vi "confocal3D.vi"() -> ()   [LabVIEW 2025]
uses:
  <vilib>/Analysis/1siggen.llb/Ramp Pattern by Samples.vi
  <vilib>/DAQmx/create/channels.llb/DAQmx Create Channel (AO-Voltage-Basic).vi
  <vilib>/DAQmx/configure/timing.llb/DAQmx Timing (Sample Clock).vi
  <vilib>/DAQmx/miscellaneous.llb/DAQmx Fill In Error Info.vi
  <vilib>/DAQmx/configure/events/hardwareSignals.llb/DAQmx Export Signal (Most Signals).vi
  <vilib>/DAQmx/read.llb/DAQmx Read (Counter 1D U32 1Chan NSamp).vi
  <vilib>/DAQmx/create/channels.llb/DAQmx Create Channel (CI-Count Edges).vi
  <vilib>/DAQmx/write.llb/DAQmx Write (Analog 1D Wfm NChan NSamp).vi
  <vilib>/DAQmx/write.llb/DAQmx Write (Analog DBL 1Chan 1Samp).vi
  <vilib>/Analysis/NI_AALBase.lvlib
panel:
  in  "step-size in microns(depth)":dbl=0.1428 format="%#_13g"
  in  "Path":path
  in  "Number of slices":i32
  in  "Enter length (nm)":dbl
  out "64bit integer":i64[](array[numeric])
  in  "pixels":dbl
  out "transposed array":dbl[][](array[numeric])
  out "Intensity Graph":dbl[][](graph)
  out "Min Voltage (V)":dbl
  out "Max Voltage (V)":dbl
  in  "Dwell time (s)":dbl
  in  "Sample mode":i32(ring)=10178 items=["Finite Samples"=10178, "Continuous Samples"=10123, "Hardware Timed Single Point"=12522]
  out "appended array":dbl[][](array[numeric])
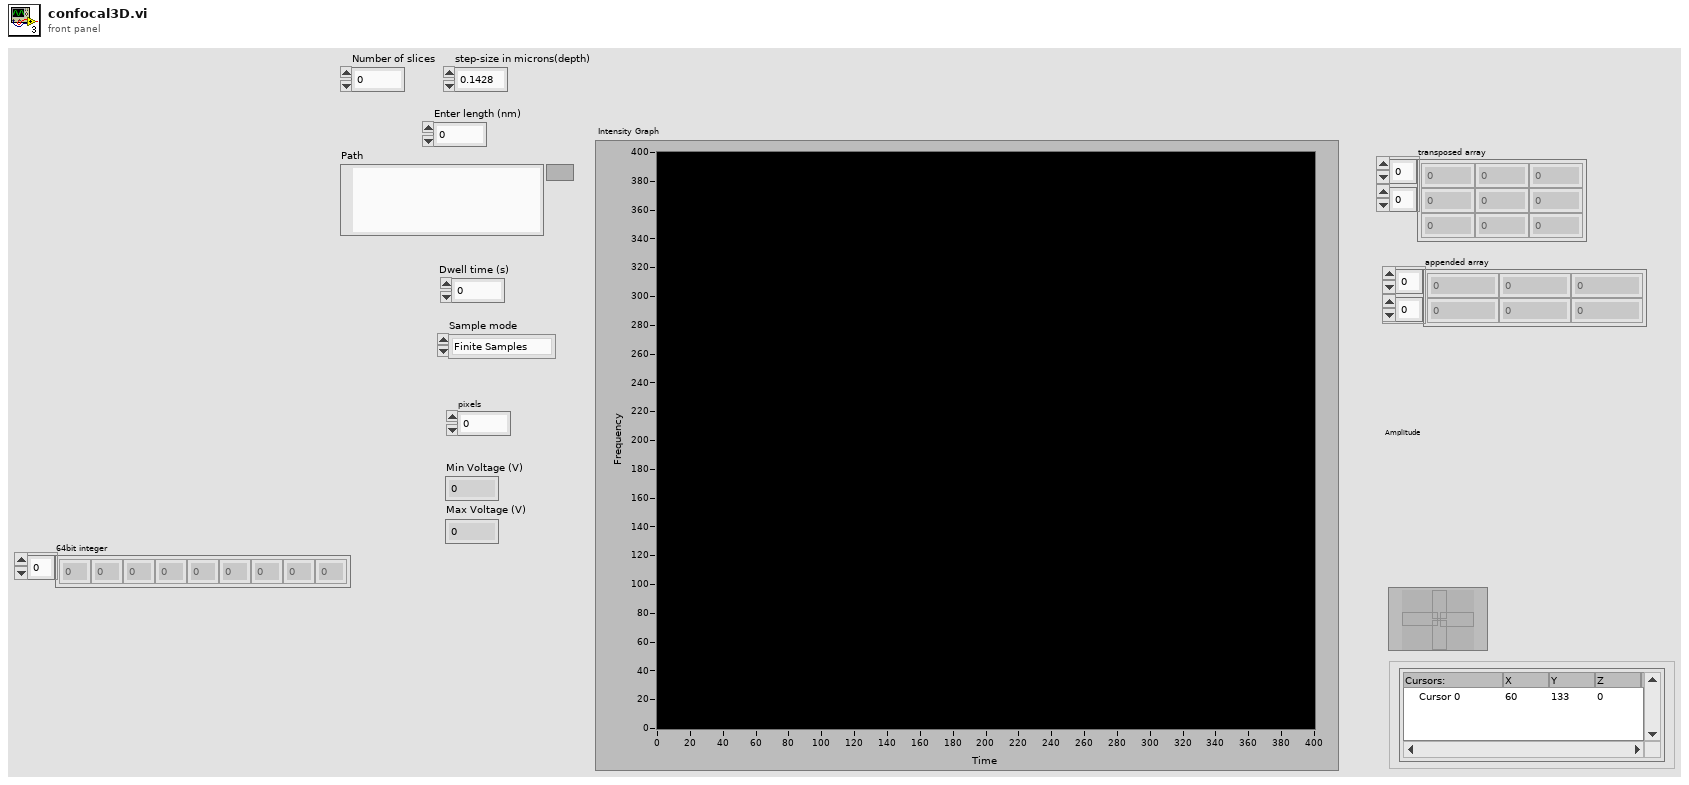
[diagram p1: front panel]
types:
  T1 = enum16{"big-endian, network order", "native, host order", "little-endian"}
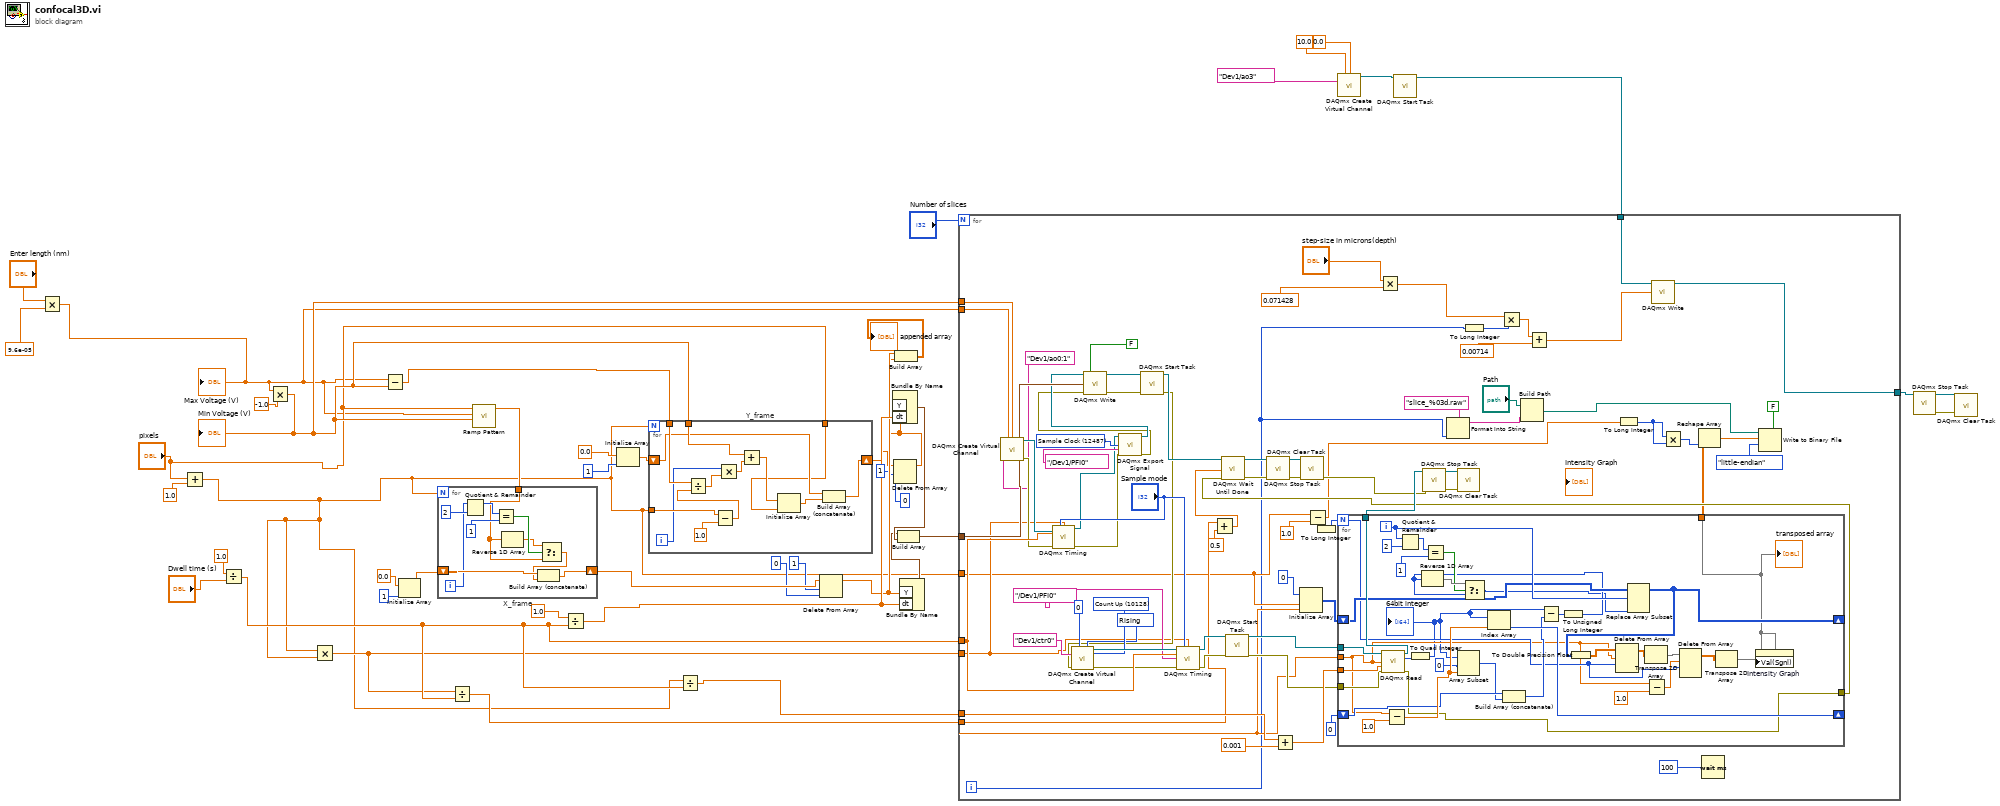
[diagram p0: block diagram]
diagram:
  n1 = Multiply(x="Enter length (nm)", y=9.6e-05) -> (x*y=w4:dbl)
  "Max Voltage (V)" <- w4
  n2 = Add(x="pixels", y=1.0) -> (x+y=w14:dbl)
  n3 = Divide(x=1.0, y="Dwell time (s)") -> (x/y=w21:dbl)
  n4 = Multiply(x=w4, y=-1.0) -> (x*y=w16:dbl)
  "Min Voltage (V)" <- w16
  n5 = Multiply(x=w14, y=w14) -> (x*y=w19:dbl)
  n6 = Subtract(x=w4, y=w16) -> (x-y=w30:dbl)
  n7 = Initialize Array(0.0 ("element"), 1 ("dimension size")) -> (w37:dbl[])
  n8 = Divide(x=w19, y=w21) -> (x/y=w18:dbl)
  n9 = call-poly <vilib>:"Ramp Pattern.vi"("start"=w16, "end"=w4, "samples"="pixels") -> ("Ramp Pattern"=w43:dbl[])  [unwired: 7 in, 1 out]
  n10 = for "X_frame" {
    N: w14 -> [_]
    shift-right: [w54] -> w29
    shift-left: w37 -> [w55]
    tunnel: w43 -> [w48]
    i -> [w49]
    n11 = Quotient & Remainder(x=w49, y=2) -> (x-y*floor(x/y)=w52:i32)  [unwired: 1 out]
    n12 = Equal?(x=w52, y=1) -> (x = y?=w50:bool)
    n13 = Reverse 1D Array(array=w48) -> (reversed array=w47:dbl[])
    n14 = Select(t=w47, s=w50, f=w48) -> (s? t:f=w46:dbl[])
    n15 = Build Array (concatenate) "Build Array"(w55, w46) -> (w54:dbl[])
  }
  n16 = Divide(x=1.0, y=w21) -> (x/y=w39:dbl)
  n17 = Initialize Array(0.0 ("element"), 1 ("dimension size")) -> (w38:dbl[])
  n18 = for "Y_frame" {
    N: w14 -> [_]
    tunnel: w14 -> [w68]
    tunnel: w30 -> [w66]
    tunnel: w16 -> [w61]
    tunnel: "pixels" -> [w56]
    shift-right: [w57] -> w25
    shift-left: w38 -> [w58]
    i -> [w63]
    n19 = Subtract(x=w68, y=1.0) -> (x-y=w65:dbl)
    n20 = Divide(x=w66, y=w65) -> (x/y=w64:dbl)
    n21 = Multiply(x=w63, y=w64) -> (x*y=w62:dbl)
    n22 = Add(x=w61, y=w62) -> (x+y=w60:dbl)
    n23 = Initialize Array(w60, w56) -> (w59:dbl[])
    n24 = Build Array (concatenate)(w58, w59) -> (w57:dbl[])
  }
  n25 = Divide(x=w14, y=w21) -> (x/y=w20:dbl)
  n26 = Delete From Array "Delete From Array"(array=w29, length=1, index=0) -> (array with subset deleted=w26:dbl[])  [unwired: 1 out]
  n27 = Delete From Array "Delete From Array"(array=w25, length=1, index=0) -> (array with subset deleted=w22:dbl[])  [unwired: 1 out]
  n28 = Bundle By Name("Y"=w22, "dt"=w39) -> (w41:waveform(dbl))  [unwired: 1 in]
  n29 = Build Array(w26, w22) -> (→"appended array":dbl[][])
  n30 = Bundle By Name("Y"=w26, "dt"=w39) -> (w40:waveform(dbl))  [unwired: 1 in]
  n31 = Build Array(w40, w41) -> (w42:waveform(dbl)[])
  n32 = call-poly <vilib>:"DAQmx Create Virtual Channel.vi"("maximum value"=10.0, "minimum value"=0.0, "physical channels"=tag "Dev1/ao3") -> ("task out"=w12:refnum<k21>)  [unwired: 11 in, 1 out]
  n33 = call <vilib>:"DAQmx Start Task.vi"("task/channels in"=w12) -> ("task out"=w11:refnum<k21>)  [unwired: 13 in, 1 out]
  n34 = for {
    N: "Number of slices" -> [_]
    tunnel: w42 -> [w131]
    tunnel: w21 -> [w117]
    tunnel: w20 -> [w114]
    tunnel: w19 -> [w99]
    tunnel: w18 -> [w98]
    tunnel: w16 -> [w95]
    tunnel: w14 -> [w93]
    tunnel: w4 -> [w92]
    tunnel: w11 -> [w90]
    tunnel: [w89] -> w8
    i -> [w81]
    w124 = 12487 items=["AI Convert Clock"=12484, "10MHz Reference Clock"=12536, "20MHz Timebase Clock"=12486, "Sample Clock"=12487, "Advance Trigger"=12488, "Reference Trigger"=12490, "Start Trigger"=12491, "Advance Complete Event"=12492, "AI Hold Complete Event"=12493, "Counter Output Event"=12494, "Change Detection Event"=12511, "Watchdog Timer Expired Event"=12512] ("signal")
    w127 = 10280 items=["Rising"=10280, "Falling"=10171] ("edge")
    w128 = 10128 items=["Count Up"=10128, "Count Down"=10124, "Externally Controlled"=10326] ("count direction")
    n35 = call-poly <vilib>:"DAQmx Create Virtual Channel.vi"("maximum value"=w92, "minimum value"=w95, "physical channels"="Dev1/ao0:1" ("Galvo mirror path")) -> ("task out"=w130:refnum<k21>, "error out"=w112:errorcluster)  [unwired: 11 in]
    n36 = call-poly <vilib>:"DAQmx Timing.vi"("task/channels in"=w130, "sample mode"="Sample mode", "samples per channel"=w99, "rate"=w117, "error in"=w112) -> ("task out"=w122:refnum<k21>, "error out"=w111:errorcluster)  [unwired: 9 in]
    n37 = call-poly <vilib>:"DAQmx Export Signal.vi"("task/channels in"=w122, "signal"=w124, "output terminal"=tag "/Dev1/PFI0", "error in"=w111) -> ("task out"=w121:refnum<k21>, "error out"=w110:errorcluster)  [unwired: 10 in]
    n38 = call-poly <vilib>:"DAQmx Write.vi"("task/channels in"=w121, "auto start"=FALSE, "data"=w131, "error in"=w110) -> ("task out"=w132:refnum<k21>, "error out"=w109:errorcluster)  [unwired: 9 in, 1 out]
    n39 = call <vilib>:"DAQmx Start Task.vi"("task/channels in"=w132, "error in"=w109) -> ("task out"=w139:refnum<k21>, "error out"=w106:errorcluster)  [unwired: 12 in]
    n40 = call-poly <vilib>:"DAQmx Create Virtual Channel.vi"("initial count"=u32 0, "count direction"=w128, "edge"=w127, "counter"="Dev1/ctr0" ("Counter path"), "error in"=w106) -> ("task out"=w134:refnum<k21>, "error out"=w108:errorcluster)  [unwired: 9 in]
    n41 = call-poly <vilib>:"DAQmx Timing.vi"("task/channels in"=w134, "sample mode"="Sample mode", "samples per channel"=w99, "rate"=w117, "source"=tag "/Dev1/PFI0", "error in"=w108) -> ("task out"=w135:refnum<k21>, "error out"=w107:errorcluster)  [unwired: 8 in]
    n42 = Add(x=w98, y=0.5) -> (x+y=w96:dbl)
    n43 = call <vilib>:"DAQmx Start Task.vi"("task/channels in"=w135, "error in"=w107) -> ("task out"=w136:refnum<k21>, "error out"=w101:errorcluster)  [unwired: 12 in]
    n44 = Add(x=w114, y=0.001) -> (x+y=w118:dbl)
    n45 = Initialize Array(u32 0 ("element"), w93, w93) -> (w138:u32[][])
    n46 = Subtract(x=w93, y=1.0) -> (x-y=w70:dbl)
    n47 = To Long Integer(number=w70) -> (32bit integer=w82:i32)
    n48 = for {
      N: w82 -> [w149]
      tunnel: w93 -> [w146]
      tunnel: w118 -> [w176]
      tunnel: w136 -> [w175]
      shift-right: [w158] -> _
      shift-left: w138 -> [w161]
      tunnel: [w170] -> w113
      shift-right: [w167] -> _
      shift-left: u64 0 ("Numeric") -> [w165]
      tunnel: w101 -> [w156]
      tunnel: [w155] -> w100
      tunnel: [w143] -> w69
      i -> [w162]
      n49 = call-poly <vilib>:"DAQmx Read.vi"("task/channels in"=w175, "number of samples per channel"=w146, "timeout"=w176, "error in"=w156) -> ("task out"=w170:refnum<k21>, "data"=w157:u32[], "error out"=w155:errorcluster)  [unwired: 9 in]
      n50 = Subtract(x=w146, y=1.0) -> (x-y=w166:dbl)
      n51 = Quotient & Remainder(x=w162, y=2) -> (x-y*floor(x/y)=w173:i32)  [unwired: 1 out]
      n52 = To Quad Integer(1:w157) -> (0:w144:i64[])
      "64bit integer" <- w144
      n53 = Equal?(x=w173, y=1) -> (x = y?=w169:bool)
      n54 = Array Subset "Array Subset"(array=w144, index=0, length=w166) -> (w145:i64[])
      n55 = Index Array "Index Array"(array=w144, index=w166) -> (element=w167:i64)
      n56 = Build Array (concatenate) "Build Array"(w165, w145) -> (w164:u64[])
      n57 = Subtract(x=w144, y=w164) -> (x-y=w163:u64[])
      n58 = To Unsigned Long Integer(number=w163) -> (unsigned 32bit integer=w160:u32[])
      n59 = Reverse 1D Array(array=w160) -> (reversed array=w171:u32[])
      n60 = Select(t=w171, s=w169, f=w160) -> (s? t:f=w159:u32[])
      n61 = Replace Array Subset "Replace Array Subset"(array=w161, new element=w159, index (row)=w162) -> (w158:u32[][])  [unwired: 1 in]
      n62 = To Double Precision Float(number=w158) -> (double precision float=w154:dbl[][])
      n63 = Delete From Array(array=w154, length=w146, index (row)=w149) -> (array with subset deleted=w153:dbl[][])  [unwired: 1 in, 1 out]
      n64 = Transpose 2D Array(2D array=w153) -> (transposed array=w152:dbl[][])
      n65 = Subtract(x=w146, y=1.0) -> (x-y=w150:dbl)
      n66 = Delete From Array(array=w152, length=w150, index (row)=w149) -> (array with subset deleted=w148:dbl[][])  [unwired: 1 in, 1 out]
      n67 = Transpose 2D Array(2D array=w148) -> (transposed array=w143:dbl[][])
      "transposed array" <- w143
      n68 = property on="Intensity Graph" class="IntGraph (strict)"("Val(Sgnl)"=w143) -> ()  [unwired: 2 in, 2 out]
    }
    n69 = call <vilib>:"DAQmx Wait Until Done.vi"("task/channels in"=w139, "timeout (sec)"=w96, "error in"=w100) -> ("task out"=w140:refnum<k21>, "error out"=w105:errorcluster)  [unwired: 11 in]
    n70 = call <vilib>:"DAQmx Stop Task.vi"("task/channels in"=w140, "error in"=w105) -> ("task out"=w133:refnum<k21>, "error out"=w104:errorcluster)  [unwired: 12 in]
    n71 = call <vilib>:"DAQmx Clear Task.vi"("task in"=w133, "error in"=w104) -> ("error out"=w103:errorcluster)  [unwired: 13 in]
    n72 = Multiply(x="step-size in microns(depth)", y=0.071428) -> (x*y=w77:dbl)
    n73 = call <vilib>:"DAQmx Stop Task.vi"("task/channels in"=w113, "error in"=w103) -> ("task out"=w141:refnum<k21>, "error out"=w102:errorcluster)  [unwired: 12 in]
    n74 = Format Into String(format string="slice_%03d.raw", w81) -> (resulting string=w83:string)  [unwired: 2 in, 1 out]
    n75 = call <vilib>:"DAQmx Clear Task.vi"("task in"=w141, "error in"=w102) -> ()  [unwired: 13 in, 1 out]
    n76 = To Long Integer(number=w81) -> (32bit integer=w80:i32)
    n77 = Multiply(x=w77, y=w80) -> (x*y=w88:dbl)
    n78 = Build Path(base path="Path", name or relative path=w83) -> (appended path=w71:path)
    n79 = Add(x=w88, y=0.00714) -> (x+y=w87:dbl)
    n80 = To Long Integer(number=w70) -> (32bit integer=w72:i32)
    n81 = call-poly <vilib>:"DAQmx Write.vi"("task/channels in"=w90, "data"=w87) -> ("task out"=w89:refnum<k21>)  [unwired: 11 in, 2 out]
    n82 = Multiply(x=w72, y=w72) -> (x*y=w74:i32)
    n83 = Reshape Array(w69, w74) -> (w76:dbl[])
    n84 = Wait (ms)(milliseconds to wait=u32 100) -> ()  [unwired: 1 out]
    n85 = Write to Binary File(file (use dialog)=w71, data=w76, 5:FALSE ("prepend array or string size? (T)"), 9:T1."little-endian" ("byte order (0:big-endian, network order)")) -> ()  [unwired: 2 in, 3 out]
  }
  n86 = call <vilib>:"DAQmx Stop Task.vi"("task/channels in"=w8) -> ("task out"=w10:refnum<k21>, "error out"=w9:errorcluster)  [unwired: 13 in]
  n87 = call <vilib>:"DAQmx Clear Task.vi"("task in"=w10, "error in"=w9) -> ()  [unwired: 13 in, 1 out]
